vi "ConfigureTrigger.vi"(8 "error in (no error)":errorcluster, 11 "IVI_Class in":refnum<class "IVI_Class.lvclass">) -> (0 "error out":errorcluster, 3 "IVI_Class out":refnum<class "IVI_Class.lvclass">)   [LabVIEW 2018, in "ScopePlugins.lvlib" / "IVI_Class.lvclass"]
uses:
  IVI_Class.lvclass
  C:/projects/ICDAS/NistPluggableModules/Scope/ScopePlugins/ScopePluginBaseClass/ScopePluginsBase.lvclass
  ScopePluginBaseClass/ScopePluginsBase.lvclass/ScopePluginsBase.ctl
  ScopePluginBaseClass/Accessors/Read Channels.vi
  <vilib>/Utility/error.llb/Error Cluster From Error Code.vi
  <vilib>/ErrorRing/Error Ring.xnode
  ScopePluginBaseClass/ScopePluginsBase.lvclass
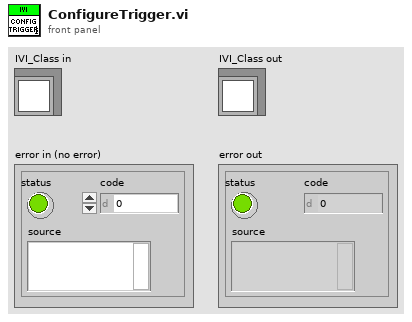
[diagram p1: front panel]
types:
  T1 = typedef "ScopePlugins.lvlib/ScopePluginsBase.lvclass/ChannelSetting(s).ctl" = cluster{"Number of Channels":i32, "Channel(s)":cluster{"Enabled":bool, "Instrument Handle":string, "Channel Name":string, "Maximum Input Frequency":dbl, "Verticle Settings":cluster{"Vertical Range":dbl, "Vertical Offset":dbl, "Probe Attenuation":dbl, "Vertical Coupling":i32}, "Connected":bool, "Input Impedance":dbl, "IO Type Instrument Handle":refnum<k15>}[]}
  T2 = typedef "ScopePlugins.lvlib/ScopePluginsBase.lvclass/TriggerSettings.ctl" = cluster{"Common Trigger Settings":cluster{"Trigger Delay":dbl, "Reference Position":dbl, "Trigger Modifier":i32, "Auto Triggered":bool}, "Specific Trigger Settings":cluster{"Source":string, "Holdoff":dbl, "Level":dbl, "Trigger Slope":enum16{"Negative", "Positive"}, "Type":enum16{"Immediate", "Edge", "Digitial", "Window", "Hysteresis", "Width", "Runt", "Glitch", "TV", "AC Line"}, "Window Mode":i32, "Low Level":dbl, "High Level":dbl, "Coupling":u16, "Hysteresis":dbl}}
  T3 = cluster{"Enabled":bool, "Instrument Handle":string, "Channel Name":string, "Maximum Input Frequency":dbl, "Verticle Settings":cluster{"Vertical Range":dbl, "Vertical Offset":dbl, "Probe Attenuation":dbl, "Vertical Coupling":i32}, "Connected":bool, "Input Impedance":dbl, "IO Type Instrument Handle":refnum<k15>}[]
  T4 = enum16{"Immediate", "Edge", "Digitial", "Window", "Hysteresis", "Width", "Runt", "Glitch", "TV", "AC Line"}
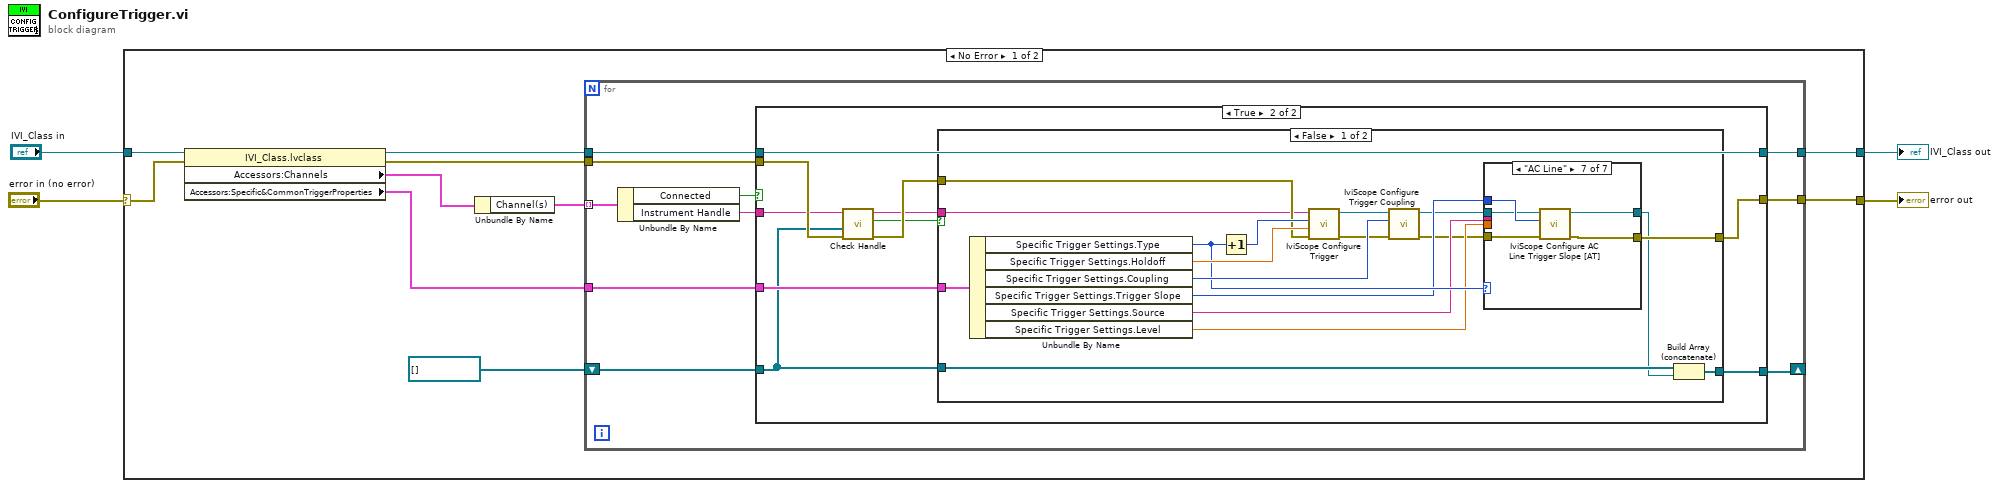
[diagram p0: block diagram]
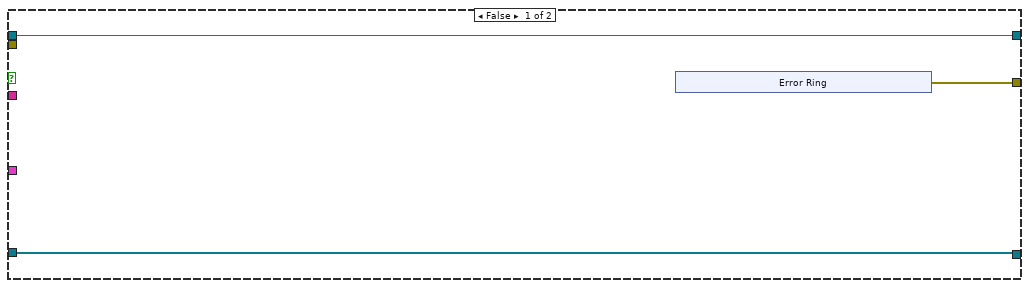
[diagram p2: hidden frame]
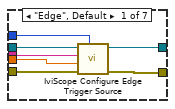
[diagram p3: hidden frame]
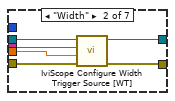
[diagram p4: hidden frame]
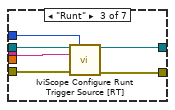
[diagram p5: hidden frame]
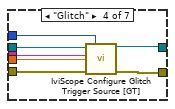
[diagram p6: hidden frame]
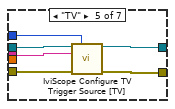
[diagram p7: hidden frame]
diagram:
  n1 = case shown="No Error" "error in (no error)" {
    selector: "error in (no error)" -> [w10 w102]
    tunnel: "IVI_Class in" -> [w14 w103]
    tunnel: [w11 w103] -> w2
    tunnel: [w13 w102] -> w1
    frame No Error {
      n2 = property class="IVI_Class.lvclass"(reference=w14, error in=w10) -> (reference out=w12:refnum<class "IVI_Class.lvclass">, error out=w9:errorcluster, "Accessors:Channels"=w8:T1, "Accessors:Specific&CommonTriggerProperties"=w7:T2)
      n3 = Unbundle By Name(w8) -> ("Channel(s)"=w6:T3)
      n4 = for {
        tunnel: w7 -> [w20]
        tunnel: w12 -> [w23]
        tunnel: [w22] -> w11
        tunnel: w9 -> [w21]
        tunnel: [w24] -> w13
        tunnel: w6 -> [w19] mode=indexing
        shift-right: [w15] -> _
        shift-left: refnum<k15>[] [] ("Array") -> [w16]
        n5 = Unbundle By Name(w19) -> ("Connected"=w18:bool, "Instrument Handle"=w17:string)
        n6 = case shown="True" w18 {
          tunnel: [w27 w41] -> w24
          tunnel: [w26 w42] -> w22
          tunnel: w23 -> [w26 w42]
          tunnel: w21 -> [_ w39]
          tunnel: w20 -> [_ w40]
          tunnel: w17 -> [_ w37]
          tunnel: w16 -> [w25 w34]
          tunnel: [w25 w33] -> w15
          frame False {
            n7 = xnode "Error Ring"() -> ("error out"=w27:errorcluster)
          }
          frame True {
            n8 = call "Check Handle.vi"("error in (no error)"=w39, "Array"=w34, "Handle In"=w37) -> ("error out"=w38:errorcluster, "Duplicate Instrument?"=w35:bool, "Handle Out"=w36:string)  [unwired: 6 in]
            n9 = case shown="False" w35 {
              tunnel: [w49 w101] -> w41
              tunnel: w40 -> [w48 _]
              tunnel: w38 -> [w47 w101]
              tunnel: w36 -> [w44 _]
              tunnel: w34 -> [w46 w100]
              tunnel: [w45 w100] -> w33
              frame False {
                n10 = Unbundle By Name(w48) -> ("Specific Trigger Settings.Type"=w55:T4, "Specific Trigger Settings.Holdoff"=w59:dbl, "Specific Trigger Settings.Coupling"=w58:u16, "Specific Trigger Settings.Trigger Slope"=w54:enum16{"Negative", "Positive"}, "Specific Trigger Settings.Source"=w53:string, "Specific Trigger Settings.Level"=w52:dbl)
                n11 = Increment(x=w55) -> (x+1=w60:T4)
                n12 = call <vilib>:"IviScope Configure Trigger.vi"("error in (no error)"=w47, "trigger holdoff (500.0 E-9 s)"=w59, "trigger type (Edge)"=w60, "instrument handle"=w44) -> ("error out"=w56:errorcluster, "instrument handle out"=w57:refnum<k15>)  [unwired: 6 in]
                n13 = call <vilib>:"IviScope Configure Trigger Coupling.vi"("error in (no error)"=w56, "trigger coupling (DC)"=w58, "instrument handle"=w57) -> ("error out"=w50:errorcluster, "instrument handle out"=w51:refnum<k15>)  [unwired: 7 in]
                n14 = case shown="\"AC Line\"" w55 {
                  tunnel: w54 -> [w66 _ w76 w85 w89 _ w99]
                  tunnel: w53 -> [w65 w72 w79 w86 w92 _ _]
                  tunnel: w52 -> [w64 w71 _ w82 _ _ _]
                  tunnel: w51 -> [w67 w73 w78 w84 w88 w93 w98]
                  tunnel: w50 -> [w63 w70 w77 w83 w87 w94 w97]
                  tunnel: [w62 w69 w74 w80 w90 w94 w96] -> w49
                  tunnel: [w61 w68 w75 w81 w91 w93 w95] -> w43
                  frame "Edge", Default {
                    n15 = call <vilib>:"IviScope Configure Edge Trigger Source.vi"("trigger slope (Positive)"=w66, "error in (no error)"=w63, "trigger level  (0.0 V)"=w64, "trigger source (CHANNEL1)"=w65, "instrument handle"=w67) -> ("error out"=w62:errorcluster, "instrument handle out"=w61:refnum<k15>)  [unwired: 5 in]
                  }
                  frame "Width" {
                    n16 = call <vilib>:"IviScope Configure Width Trigger Source [WT].vi"("error in (no error)"=w70, "trigger level (0.0 V)"=w71, "trigger source (\"CHANNEL1\")"=w72, "instrument handle"=w73) -> ("error out"=w69:errorcluster, "instrument handle out"=w68:refnum<k15>)  [unwired: 6 in]
                  }
                  frame "Runt" {
                    n17 = call <vilib>:"IviScope Configure Runt Trigger Source [RT].vi"("instrument handle"=w78, "runt polarity (Positive)"=w76, "trigger source (\"CHANNEL1\")"=w79, "error in (no error)"=w77) -> ("instrument handle out"=w75:refnum<k15>, "error out"=w74:errorcluster)  [unwired: 10 in]
                  }
                  frame "Glitch" {
                    n18 = call <vilib>:"IviScope Configure Glitch Trigger Source [GT].vi"("instrument handle"=w84, "glitch polarity (Positive)"=w85, "trigger source (\"CHANNEL1\")"=w86, "trigger level (0.0 V)"=w82, "error in (no error)"=w83) -> ("instrument handle out"=w81:refnum<k15>, "error out"=w80:errorcluster)  [unwired: 9 in]
                  }
                  frame "TV" {
                    n19 = call <vilib>:"IviScope Configure TV Trigger Source [TV].vi"("instrument handle"=w88, "tv trigger polarity (Positive)"=w89, "trigger source (\"CHANNEL1\")"=w92, "error in (no error)"=w87) -> ("instrument handle out"=w91:refnum<k15>, "error out"=w90:errorcluster)  [unwired: 10 in]
                  }
                  frame "Immediate" {
                  }
                  frame "AC Line" {
                    n20 = call <vilib>:"IviScope Configure AC Line Trigger Slope [AT].vi"("error in (no error)"=w97, "ac line trigger slope (Positive)"=w99, "instrument handle"=w98) -> ("error out"=w96:errorcluster, "instrument handle out"=w95:refnum<k15>)  [unwired: 7 in]
                  }
                }
                n21 = Build Array (concatenate)(w46, w43) -> (w45:refnum<k15>[])
              }
              frame True {
              }
            }
          }
        }
      }
    }
    frame Error {
    }
  }
  "error out" <- w1
  "IVI_Class out" <- w2
